vi "Target_0505.vi"() -> ()   [LabVIEW 2018]
uses:
  <vilib>/Platform/TimedLoop/XDataNode/timing_clust.ctl
  <vilib>/Platform/TimedLoop/XDataNode/nitl_modes.ctl
  <vilib>/Platform/TimedLoop/XDataNode/wakeup.ctl
  <vilib>/rvi/eio/common/nirviEmuTemplateMethod_errors.vi
  <vilib>/rvi/Emulation/niFpgaGetClockAttributes.vi
  <vilib>/rvi/Emulation/niFpgaSctlEmulationGetInTimedLoop.vi
  <vilib>/rvi/Emulation/niFpgaEmulationReportErrorSimple.vi
  <vilib>/rvi/Emulation/niFpgaProcessEmulError.vi
  <vilib>/rvi/Emulation/niFpgaCriticalErrorInLSC.vi
  <vilib>/rvi/Memory/Memory_Emulation/niFpgaMemoryFastEmulationDramWriteAndRequestData.vi
  <vilib>/rvi/Memory/Memory_Emulation/niFpgaMemoryEmulationDramWriteAndRequestData.vi
  <vilib>/rvi/DataTransferAndStorage/Container/Common/niFpgaContainerGetUniqueNameForEmu.vi
  <vilib>/rvi/Memory/Memory_Emulation/niFpgaMemoryEmulationDramWriteAndRequestDataApplyByteEnables.vi
  <vilib>/rvi/interface/RandomDataEmulation/niFpgaRandomDataHandleErrors.vi
  <vilib>/rvi/Memory/Memory_Emulation/nirvimemoryFastEmulation.vi
  <vilib>/rvi/Memory/Memory_Emulation/nirvimemoryEmulation.vi
  <vilib>/rvi/Emulation/niFpgaEmulationIsFPGAContextNoSignature.vi
  <vilib>/rvi/errors/nirviReportUnexpectedCaseInternalError (U32).vi
  <vilib>/rvi/Memory/Memory_Emulation/niFpgaMemoryEmulationCacheClearOnFirstRun.vi
  <vilib>/rvi/Memory/Memory_Emulation/nirvimemoryEmulationManagerCache_MakeExclusive.vi
  <vilib>/rvi/Memory/Memory_Emulation/niFpgaMemoryEmulationValidateCache.vi
  <vilib>/rvi/Memory/Memory_Emulation/nirvimemoryEmulationManagerCache_InsertValue.vi
  <vilib>/Utility/error.llb/Clear Errors.vi
  <vilib>/rvi/Memory/Memory_Emulation/nirvimemoryEmulationManagerCache_ReleaseExclusive.vi
  <vilib>/rvi/Memory/Memory_Emulation/nirvimemoryEmulationManagerCache_GetValue.vi
  <vilib>/rvi/Memory/Memory_Emulation/nirvimemoryEmulationManagerCache_SetValue.vi
  <vilib>/rvi/Emulation/niFpgaSctlEmulationResourceMgr.vi
  <vilib>/eio/EIONode/EIONode.xnode
  <vilib>/Platform/TimedLoop/XDataNode/XDataNode.xnode
  <vilib>/rvi/DataTransferAndStorage/Container/XNode/niFpgaContainer.xnode
  <vilib>/rvi/Memory/Memory_Emulation/niFpgaMemoryEmulationDramRetrieveData.vi
  <vilib>/rvi/interface/RandomDataEmulation/nirviRandomDataFpgaReadWriteTemplate.vi
  <vilib>/Platform/TimedLoop/XDataNode/XDNodeRunTimeDep.lvlib
  <instrlib>/_niInstr/Basic Elements/v1/FPGA/niInstr Basic Elements v1 FPGA.lvlib
panel:
  in  "Хватит":bool
  in  "48":bool[](array[boolean])=[FALSE, FALSE, FALSE, FALSE, FALSE, FALSE, FALSE, FALSE, FALSE, FALSE, FALSE, FALSE, FALSE, FALSE, FALSE, FALSE, FALSE, FALSE, FALSE, FALSE, FALSE, FALSE, FALSE, FALSE, FALSE, FALSE, FALSE, FALSE, FALSE, FALSE, FALSE, FALSE, FALSE, FALSE, FALSE, FALSE, FALSE, FALSE, FALSE, FALSE, FALSE, FALSE, FALSE, FALSE, FALSE, FALSE, FALSE, FALSE]
  in  "48":u8=48
  out "Записали адресов":u32
  in  "3445760":u32=3445760
  in  "20":u8=20
  in  "Стоп":bool
  out "SPI_OFF":bool
  in  "12 2":u8=12
  in  "FR":u8=19
  in  "19":u8=19
  in  "SPI":bool
  in  "W(T)/R(F)":bool
  in  "Адрес":u8
  in  "Кол-во":u16=256
  in  "256":u16=256
  in  "258":u16=258
  in  "255":u16=255
  in  "Upd_RD":bool
  in  "Upd_WR":bool
  in  "SYS_RST_N":bool
  in  "Автомат":bool
  in  "Кадр в память":bool
  in  "Кадр на ПК":bool
  in  "Нач_адр":u32
  in  "Кон_адр":u32=26920
  out "Записали FIFO":bool
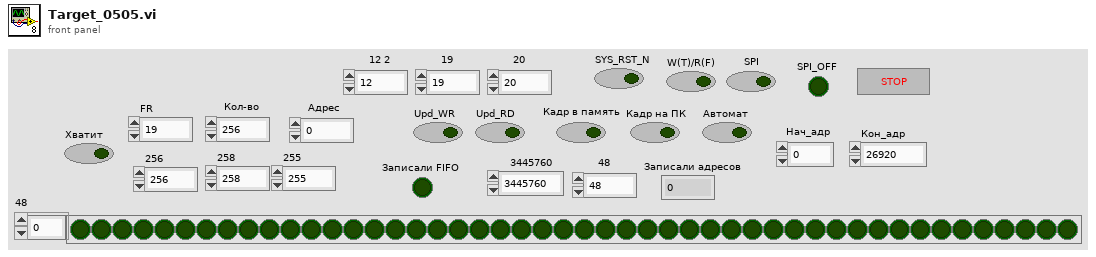
[diagram p1: front panel]
types:
  T1 = typedef "XDNodeRunTimeDep.lvlib/timing_clust.ctl" = cluster{"Expected End [f-1]":u64, "Actual End [f-1]":u64, "Finished Late? [f-1]":bool, "Expected End [i-1]":u64, "Actual End [i-1]":u64, "Finished Late? [i-1]":bool, "Expected Start [i]":u64, "Actual Start [i]":u64, "Expected Start [f]":u64, "Actual Start [f]":u64, "Source Name":string, "Structure Name":string, "Period":i64, "Deadline":i64, "Offset":i64, "Start":i64, "Priority":i32, "Timeout":i32, "Mode":T2, "Wakeup Reason":T3, "Error":errorcluster, "Source Type":string, "Secondary Source Type":string, "Global End Time":u64, "Global Start Time":u64, "Frame Duration":u64, "Iteration Duration":u64, "Assigned CPU":i32, "I/O Scan Engine Mode":u32}
  T2 = typedef "XDNodeRunTimeDep.lvlib/nitl_modes.ctl" = enum32{"No Change", "Process missed periods, maintain original phase", "Discard missed periods, maintain original phase", "Process missed periods, ignore original phase", "Discard missed periods, ignore original phase"}
  T3 = typedef "XDNodeRunTimeDep.lvlib/wakeup.ctl" = enum32{"Normal", "Aborted", "Asynchronous wakeup", "Timing source error", "Timed loop error", "Timeout"}
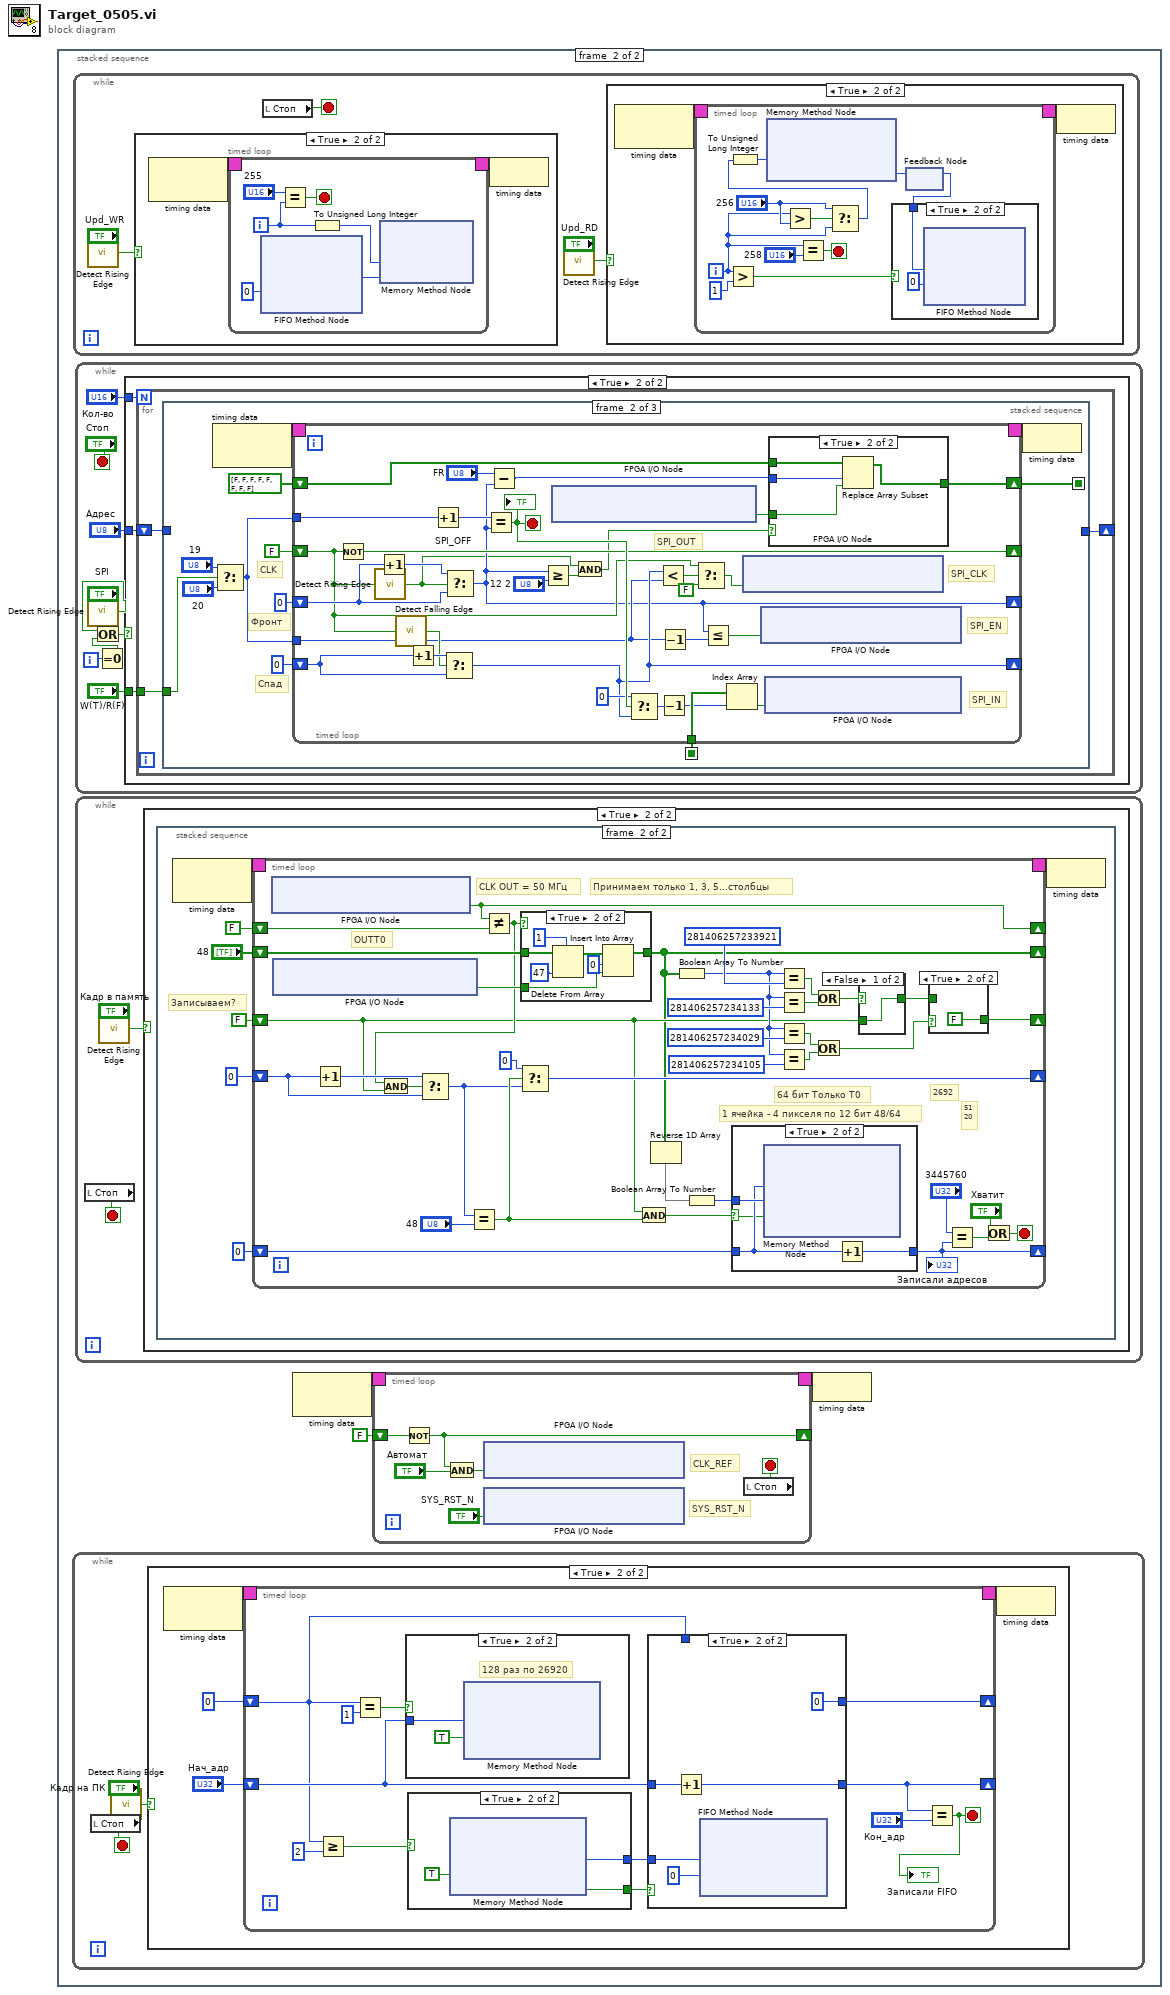
[diagram p0: block diagram]
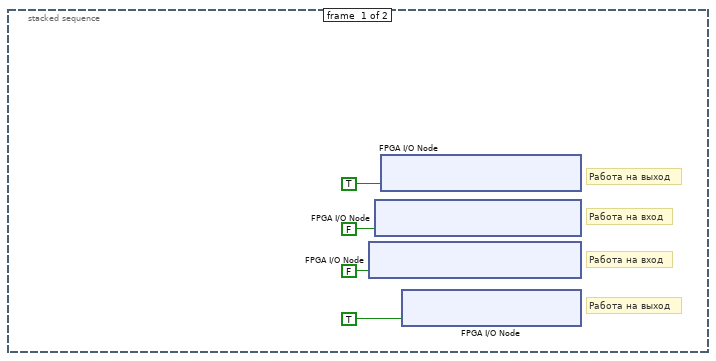
[diagram p2: hidden frame]
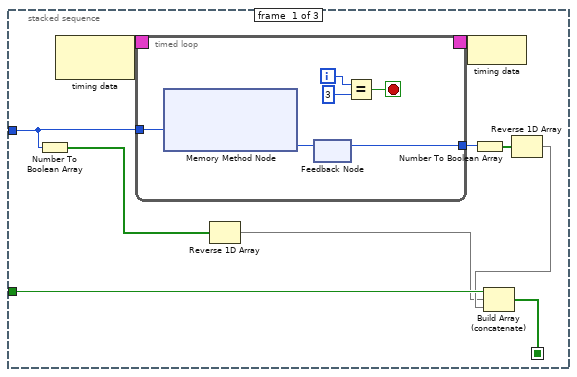
[diagram p4: hidden frame]
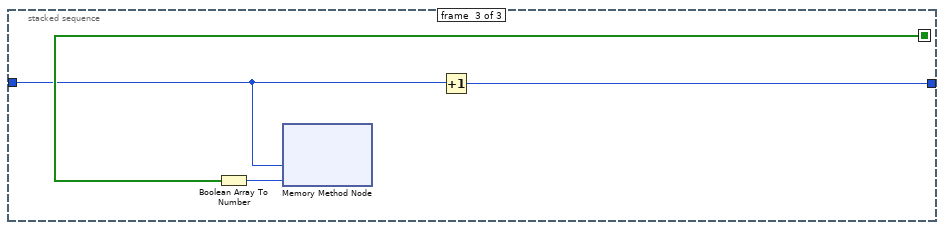
[diagram p6: hidden frame]
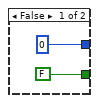
[diagram p11: hidden frame]
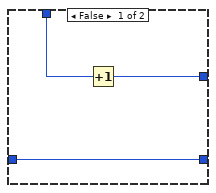
[diagram p13: hidden frame]
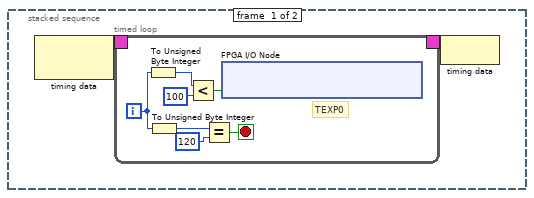
[diagram p15: hidden frame]
diagram:
  n1 = stacked-sequence {
    frame #0 {
      # "Работа на выход"
      # "Работа на вход"
      # "Работа на вход"
      # "Работа на выход"
      n2 = xnode "FPGA I/O Node"("IO Module\\DDCA_DIO16-23_WE"=FALSE ("IO Module\\DDCA_DIO16-23_WE")) -> ()  [unwired: 1 in, 1 out]
      n3 = xnode "FPGA I/O Node"("IO Module\\DDCA_DIO8-15_WE"=FALSE ("IO Module\\DDCA_DIO8-15_WE")) -> ()  [unwired: 1 in, 1 out]
      n4 = xnode "FPGA I/O Node"("IO Module\\DDCA_DIO0-7_WE"=TRUE ("IO Module\\DDCA_DIO0-7_WE")) -> ()  [unwired: 1 in, 1 out]
      n5 = xnode "FPGA I/O Node"("IO Module\\DDCA_PFI_WE"=TRUE ("IO Module\\DDCA_DIO16-23_WE")) -> ()  [unwired: 1 in, 1 out]
    }
    frame #1 {
      n6 = while {
        stop <- w148 stop-if-true
        n7 = local read "Стоп"() -> (w148:bool)
        n8 = call <instrlib>:"Detect Rising Edge.vi"("signal"="Кадр на ПК") -> ("edge detected"=w147:bool)  [unwired: 14 in]
        n9 = case shown="True" w147 {
          frame False {
          }
          frame True {
            n10 = node-c288() -> (w152:T1)  [unwired: 1 in]
            n11 = timed-loop {
              shift-right: [w163] -> _
              shift-left: "Нач_адр" -> [w157]
              timing: w152 -> [_]
              timing-out: [_] -> w151
              shift-right: [w155] -> _
              shift-left: u8 0 -> [w156]
              stop <- w164 stop-if-true
              n12 = Greater Or Equal?(x=w156, y=u8 2 ("2")) -> (x >= y?=w158:bool)
              n13 = Equal?(x=w156, y=u8 1 ("1")) -> (x = y?=w161:bool)
              n14 = case shown="True" w161 {
                tunnel: w157 -> [_ w171]
                frame False {
                }
                frame True {
                  # "128 раз по 26920"
                  n15 = xnode ("Memory Method Node")("Address"=w171, "Input Valid"=TRUE) -> ()  [unwired: 1 in, 2 out]
                }
              }
              n16 = case shown="True" w158 {
                tunnel: [u8 0 ("Data") w169] -> w162
                tunnel: [FALSE ("Output Valid") w168] -> w153
                frame False {
                }
                frame True {
                  n17 = xnode ("Memory Method Node")("Ready for Output"=TRUE ("Ready For Output")) -> ("Data"=w169:u64, "Output Valid"=w168:bool)  [unwired: 1 in, 1 out]
                }
              }
              n18 = case shown="True" w153 {
                tunnel: [w172 w179] -> w163
                tunnel: w162 -> [_ w176]
                tunnel: w157 -> [w172 w178]
                tunnel: w156 -> [w174 _]
                tunnel: [w173 u8 0] -> w155
                frame False {
                  n19 = Increment(x=w174) -> (x+1=w173:u8)
                }
                frame True {
                  n20 = Increment(x=w178) -> (x+1=w179:u32)
                  n21 = xnode ("FIFO Method Node")("Element"=w176, "Timeout"=u8 0) -> ()  [unwired: 1 in, 2 out]
                }
              }
              n22 = Equal?(x=w163, y="Кон_адр") -> (x = y?=w164:bool)
              "Записали FIFO" <- w164
            }
            n23 = node-c288(w151) -> ()
          }
        }
      }
      n24 = while {
        stop <- w104 stop-if-true
        n25 = call <instrlib>:"Detect Rising Edge.vi"("signal"="Upd_WR") -> ("edge detected"=w102:bool)  [unwired: 14 in]
        n26 = case shown="True" w102 {
          frame False {
          }
          frame True {
            n27 = node-c288() -> (w125:T1)  [unwired: 1 in]
            n28 = timed-loop {
              timing: w125 -> [_]
              timing-out: [_] -> w124
              i -> [w128]
              stop <- w126 stop-if-true
              n29 = xnode ("FIFO Method Node")("Timeout"=0) -> ("Element"=w131:u8)  [unwired: 1 in, 2 out]
              n30 = Equal?(x="255", y=w128) -> (x = y?=w126:bool)
              n31 = To Unsigned Long Integer(number=w128) -> (unsigned 32bit integer=w130:u32)
              n32 = xnode ("Memory Method Node")("Address"=w130, "Data"=w131) -> ()  [unwired: 1 in, 1 out]
            }
            n33 = node-c288(w124) -> ()
          }
        }
        n34 = local read "Стоп"() -> (w104:bool)
        n35 = call <instrlib>:"Detect Rising Edge.vi"("signal"="Upd_RD") -> ("edge detected"=w100:bool)  [unwired: 14 in]
        n36 = case shown="True" w100 {
          frame False {
          }
          frame True {
            n37 = node-c288() -> (w106:T1)  [unwired: 1 in]
            n38 = timed-loop {
              timing: w106 -> [_]
              timing-out: [_] -> w105
              i -> [w109]
              stop <- w112 stop-if-true
              n39 = Greater?(x=w109, y=u8 1) -> (0:w116:bool)
              n40 = Greater?(x=w109, y="256") -> (0:w111:bool)
              n41 = Equal?(x=w109, y="258") -> (x = y?=w112:bool)
              n42 = Select(t="256", s=w111, f=w109) -> (s? t:f=w108:i32)
              n43 = To Unsigned Long Integer(number=w108) -> (unsigned 32bit integer=w115:u32)
              n44 = xnode ("Memory Method Node")("Address"=w115) -> ("Data"=w114:u8)  [unwired: 2 in, 2 out]
              n45 = feedback #1() -> (w107:u8)  [unwired: 1 in]
              n46 = case shown="True" w116 {
                tunnel: w107 -> [_ w118]
                frame False {
                }
                frame True {
                  n47 = xnode ("FIFO Method Node")("Element"=w118, "Timeout"=u8 0) -> ()  [unwired: 1 in, 2 out]
                }
              }
              n48 = feedback-in #1(w114) -> ()
            }
            n49 = node-c288(w105) -> ()
          }
        }
      }
      n50 = while {
        i -> [w10]
        stop <- "Стоп" stop-if-true
        n51 = call <instrlib>:"Detect Rising Edge.vi"("signal"="SPI") -> ("edge detected"=w8:bool)  [unwired: 14 in]
        n52 = Equal To 0?(x=w10) -> (x = 0?=w9:bool)
        n53 = Or(x=w8, y=w9) -> (x .or. y?=w11:bool)
        n54 = case shown="True" w11 {
          tunnel: "W(T)/R(F)" -> [_ w19]
          tunnel: "Адрес" -> [_ w18]
          tunnel: "Кол-во" -> [_ w17]
          frame False {
          }
          frame True {
            n55 = for {
              N: w17 -> [_]
              tunnel: w19 -> [w22]
              shift-right: [w20] -> _
              shift-left: w18 -> [w21]
              n56 = stacked-sequence {
                seq-local: [w26 _ _] -> [_ w50 _]
                seq-local: [_ w48 _] -> [_ _ w98]
                tunnel: w22 -> [w28 w46 _]
                tunnel: w21 -> [w25 _ w96]
                tunnel: [_ _ w99] -> w20
                frame #0 {
                  n57 = Number To Boolean Array(number=w25) -> (Boolean array=w23:bool[])
                  n58 = node-c288() -> (w32:T1)  [unwired: 1 in]
                  n59 = timed-loop {
                    timing: w32 -> [_]
                    timing-out: [_] -> w31
                    tunnel: w25 -> [w38]
                    tunnel: [w36] -> w30
                    i -> [w35]
                    stop <- w33 stop-if-true
                    n60 = xnode ("Memory Method Node")("Address"=w38) -> ("Data"=w37:u8)  [unwired: 1 in, 1 out]
                    n61 = feedback-in #2(w37) -> ()
                    n62 = feedback #2() -> (w36:u8)  [unwired: 1 in]
                    n63 = Equal?(x=w35, y=u8 3) -> (x = y?=w33:bool)
                  }
                  n64 = Reverse 1D Array(array=w23) -> (reversed array=w24:bool[])
                  n65 = node-c288(w31) -> ()
                  n66 = Number To Boolean Array(number=w30) -> (Boolean array=w29:bool[])
                  n67 = Reverse 1D Array(array=w29) -> (reversed array=w27:bool[])
                  n68 = Build Array (concatenate)(w28, w24, w27) -> (w26:bool[])
                }
                frame #1 {
                  # "Фронт"
                  # "Спад"
                  # "CLK"
                  n69 = node-c288() -> (w54:T1)  [unwired: 1 in]
                  n70 = Select(t="19", s=w46, f="20") -> (s? t:f=w45:u8)
                  n71 = timed-loop {
                    timing: w54 -> [_]
                    timing-out: [_] -> w53
                    shift-right: [w66] -> _
                    shift-left: FALSE -> [w65]
                    shift-right: [w71] -> _
                    shift-left: u8 0 -> [w74]
                    shift-right: [w59] -> _
                    shift-left: u8 0 -> [w85]
                    tunnel: w45 -> [w60]
                    tunnel: w45 -> [w76]
                    tunnel: w50 -> [w70]
                    shift-right: [w67] -> w48
                    shift-left: bool[] [FALSE, FALSE, FALSE, FALSE, FALSE, FALSE, FALSE, FALSE] -> [w68]
                    stop <- w73 stop-if-true
                    # "SPI_OUT"
                    # "SPI_IN"
                    # "SPI_CLK"
                    # "SPI_EN"
                    n72 = Not(x=w65) -> (.not. x?=w66:bool)
                    n73 = call <instrlib>:"Detect Rising Edge.vi"("signal"=w65) -> ("edge detected"=w57:bool)  [unwired: 14 in]
                    n74 = Increment(x=w85) -> (x+1=w86:u8)
                    n75 = call <instrlib>:"Detect Falling Edge.vi"("signal"=w65) -> ("edge detected"=w75:bool)  [unwired: 14 in]
                    n76 = Increment(x=w74) -> (x+1=w84:u8)
                    n77 = Increment(x=w76) -> (x+1=w77:u8)
                    n78 = Select(t=w84, s=w75, f=w74) -> (s? t:f=w71:u8)
                    n79 = Select(t=w86, s=w57, f=w85) -> (s? t:f=w59:u8)
                    n80 = Equal?(x=w77, y=w59) -> (x = y?=w73:bool)
                    "SPI_OFF" <- w73
                    n81 = Subtract(x="FR", y=w59) -> (x-y=w64:u8)
                    n82 = Greater Or Equal?(x=w59, y="12 2") -> (x >= y?=w58:bool)
                    n83 = xnode "FPGA I/O Node"() -> ("IO Module\\DDCA_DIO19_Read"=w79:bool)  [unwired: 1 in, 1 out]
                    n84 = And(x=w57, y=w58) -> (x .and. y?=w56:bool)
                    n85 = Select(t=u8 0, s=w73, f=w71) -> (s? t:f=w63:u8)
                    n86 = Less?(x=w71, y=w60) -> (x < y?=w82:bool)
                    n87 = Decrement(x=w63) -> (x-1=w62:u8)
                    n88 = Decrement(x=w60) -> (x-1=w61:u8)
                    n89 = Select(t=w65, s=w82, f=FALSE) -> (s? t:f=w80:bool)
                    n90 = Less Or Equal?(x=w59, y=w61) -> (x <= y?=w83:bool)
                    n91 = Index Array(array=w70, index=w62) -> (element=w69:bool)
                    n92 = xnode "FPGA I/O Node"("IO Module\\DDCA_DIO2_Write"=w80) -> ()  [unwired: 1 in, 1 out]
                    n93 = xnode "FPGA I/O Node"("IO Module\\DDCA_DIO3_Write"=w83) -> ()  [unwired: 1 in, 1 out]
                    n94 = xnode "FPGA I/O Node"("IO Module\\DDCA_PFI2_Write"=w69) -> ()  [unwired: 1 in, 1 out]
                    n95 = case shown="True" w56 {
                      tunnel: w79 -> [_ w90]
                      tunnel: w64 -> [_ w88]
                      tunnel: w68 -> [w87 w91]
                      tunnel: [w87 w89] -> w67
                      frame False {
                      }
                      frame True {
                        n96 = Replace Array Subset(array=w91, new element=w90, index=w88) -> (w89:bool[])
                      }
                    }
                  }
                  n97 = node-c288(w53) -> ()
                }
                frame #2 {
                  n98 = Boolean Array To Number(Boolean array=w98) -> (number=w97:u8)
                  n99 = xnode ("Memory Method Node")("Address"=w96, "Data"=w97) -> ()  [unwired: 2 in, 2 out]
                  n100 = Increment(x=w96) -> (x+1=w99:u8)
                }
              }
            }
          }
        }
      }
      n101 = while {
        stop <- w186 stop-if-true
        n102 = local read "Стоп"() -> (w186:bool)
        n103 = call <instrlib>:"Detect Rising Edge.vi"("signal"="Кадр в память") -> ("edge detected"=w185:bool)  [unwired: 14 in]
        n104 = case shown="True" w185 {
          frame False {
          }
          frame True {
            n105 = stacked-sequence {
              frame #0 {
                n106 = node-c288() -> (w188:T1)  [unwired: 1 in]
                n107 = timed-loop {
                  timing: w188 -> [_]
                  timing-out: [_] -> w187
                  i -> [w190]
                  stop <- w192 stop-if-true
                  # "TEXP0"
                  n108 = To Unsigned Byte Integer(number=w190) -> (unsigned 8bit integer=w191:u8)
                  n109 = To Unsigned Byte Integer(number=w190) -> (unsigned 8bit integer=w189:u8)
                  n110 = Less?(x=w191, y=u8 100) -> (x < y?=w193:bool)
                  n111 = Equal?(x=w189, y=u8 120) -> (x = y?=w192:bool)
                  n112 = xnode "FPGA I/O Node"("IO Module\\DDCA_DIO4_Write"=w193) -> ()  [unwired: 1 in, 1 out]
                }
                n113 = node-c288(w187) -> ()
              }
              frame #1 {
                # "Записываем?"
                n114 = node-c288() -> (w206:T1)  [unwired: 1 in]
                n115 = timed-loop {
                  shift-right: [w211] -> _
                  shift-left: FALSE -> [w243]
                  shift-right: [w213] -> _
                  shift-left: "48" -> [w240]
                  timing: w206 -> [_]
                  timing-out: [_] -> w205
                  shift-right: [w241] -> _
                  shift-left: u32 0 -> [w242]
                  shift-right: [w229] -> _
                  shift-left: FALSE -> [w216]
                  shift-right: [w219] -> _
                  shift-left: u8 0 -> [w222]
                  stop <- w210 stop-if-true
                  # "5120"
                  # "2692"
                  # "Принимаем только 1, 3, 5...столбцы"
                  # "OUTT0"
                  # "CLK OUT = 50 МГц"
                  # "1 ячейка - 4 пикселя по 12 бит 48/64"
                  # "64 бит Только T0"
                  n116 = xnode "FPGA I/O Node"() -> ("IO Module\\DDCA_DIO9_Read"=w211:bool)  [unwired: 1 in, 1 out]
                  n117 = xnode "FPGA I/O Node"() -> ("IO Module\\DDCA_DIO11_Read"=w239:bool)  [unwired: 1 in, 1 out]
                  n118 = Increment(x=w222) -> (x+1=w223:u8)
                  n119 = Not Equal?(x=w211, y=w243) -> (x != y?=w217:bool)
                  n120 = And(x=w217, y=w216) -> (x .and. y?=w215:bool)
                  n121 = Select(t=w223, s=w215, f=w222) -> (s? t:f=w218:u8)
                  n122 = Equal?(x=w218, y="48") -> (x = y?=w221:bool)
                  n123 = Select(t=u8 0, s=w221, f=w218) -> (s? t:f=w219:u8)
                  n124 = case shown="True" w217 {
                    tunnel: w240 -> [w253 w256]
                    tunnel: w239 -> [_ w259]
                    tunnel: [w253 w258] -> w213
                    frame False {
                    }
                    frame True {
                      n125 = Delete From Array(array=w256, length=u8 1, index=u8 47) -> (array with subset deleted=w257:bool[])  [unwired: 1 out]
                      n126 = Insert Into Array(array=w257, index=u8 0, new element=w259) -> (w258:bool[])
                    }
                  }
                  n127 = And(x=w216, y=w221) -> (x .and. y?=w224:bool)
                  n128 = Reverse 1D Array(array=w213) -> (reversed array=w212:bool[])
                  n129 = Boolean Array To Number(Boolean array=w213) -> (number=w226:u64)
                  n130 = Boolean Array To Number(Boolean array=w212) -> (number=w214:u64)
                  n131 = case shown="True" w224 {
                    selector: w224 -> [_ w245]
                    tunnel: [w244 w248] -> w241
                    tunnel: w214 -> [_ w247]
                    tunnel: w242 -> [w244 w246]
                    frame False {
                    }
                    frame True {
                      n132 = xnode ("Memory Method Node")("Address"=w246, "Data"=w247, "Input Valid"=w245) -> ()  [unwired: 1 in, 2 out]
                      n133 = Increment(x=w246) -> (x+1=w248:u32)
                    }
                  }
                  "Записали адресов" <- w241
                  n134 = Equal?(x=w226, y=u64 281406257233921 ("SOF")) -> (x = y?=w236:bool)
                  n135 = Equal?(x=w226, y=u64 281406257234133 ("SOL")) -> (x = y?=w235:bool)
                  n136 = Equal?(x=w226, y=u64 281406257234029 ("EOL")) -> (x = y?=w233:bool)
                  n137 = Equal?(x=w226, y=u64 281406257234105 ("EOF")) -> (x = y?=w232:bool)
                  n138 = Or(x=w236, y=w235) -> (x .or. y?=w234:bool)
                  n139 = Or(x=w233, y=w232) -> (x .or. y?=w231:bool)
                  n140 = case shown="False" w234 {
                    selector: w234 -> [_ w252]
                    tunnel: [w251 w252] -> w230
                    tunnel: w216 -> [w251 _]
                    frame False {
                    }
                    frame True {
                    }
                  }
                  n141 = case shown="True" w231 {
                    tunnel: [w249 FALSE] -> w229
                    tunnel: w230 -> [w249 _]
                    frame False {
                    }
                    frame True {
                    }
                  }
                  n142 = Equal?(x="3445760", y=w241) -> (x = y?=w208:bool)
                  n143 = Or(x="Хватит", y=w208) -> (x .or. y?=w210:bool)
                }
                n144 = node-c288(w205) -> ()
              }
            }
          }
        }
      }
      n145 = node-c288() -> (w7:T1)  [unwired: 1 in]
      n146 = timed-loop {
        timing: w7 -> [_]
        timing-out: [_] -> w6
        shift-right: [w136] -> _
        shift-left: FALSE -> [w140]
        stop <- w141 stop-if-true
        # "SYS_RST_N"
        # "CLK_REF"
        n147 = Not(x=w140) -> (.not. x?=w136:bool)
        n148 = And(x=w136, y="Автомат") -> (x .and. y?=w137:bool)
        n149 = xnode "FPGA I/O Node"("IO Module\\DDCA_DIO1_Write"=w137) -> ()  [unwired: 1 in, 1 out]
        n150 = xnode "FPGA I/O Node"("IO Module\\DDCA_DIO0_Write"="SYS_RST_N") -> ()  [unwired: 1 in, 1 out]
        n151 = local read "Стоп"() -> (w141:bool)
      }
      n152 = node-c288(w6) -> ()
    }
  }
